vi "Tank Data Global.vi"(0 "Tank Data IN":dbl[](array[numeric]), 1 "Pump Data Mode":T4, 5 "Tank Temp Variables":T3, 7 "Watlow Present":bool, 9 "Pressure Offsets":dbl[](array[numeric])=[0.0, 0.0, 0.0, 0.0, 0.0, 0.0], 11 "Cal Coefficients":dbl[][](array[numeric]), 12 "Intitial Times":dbl[](array[numeric]), 13 "Pumps Present":bool[](array[boolean])) -> (4 "Tank Data OUT":dbl[](array[numeric]), 6 "Pump Data":T2={"Voltages"=[0.015201568603515625, 0.00335693359375, 0.003021240234375, 0.12260055541992188, 0.06085968017578125, 0.052234649658203125], "PumpCurrent"=[0.015201568603515625, 0.00335693359375, 0.003021240234375, 0.12260055541992188, 0.06085968017578125, 0.052234649658203125], "Speed"=[0.0, 0.0, 0.0, 0.0, 0.0, 0.0], "ControllerCurrent"=[0.015201568603515625, 0.00335693359375, 0.003021240234375, 0.12260055541992188, 0.06085968017578125, 0.052234649658203125], "Pressure"=[0.015201568603515625, 0.00335693359375, 0.003021240234375, 0.12260055541992188, 0.06085968017578125, 0.052234649658203125], "Flow"=[0.0, 0.0, 0.0, 0.125, 0.0625, 0.0625], "Elapsed Time (Display)"=[7.1, 7.1, 7.1, 458133.45, 458138.85000000003, 458126.75], "Avg Pressure"=0.0, "Avg Speed"=0.0, "Elapsed Time"=[4074.9003000000002, 4074.9003000000002, 4074.9003000000002, 4074.9003000000002, 4074.9003000000002, 4074.9003000000002]} {"Elapsed Time" format="%<%H:%M:%S>t"; "Elapsed Time (Display)" format="%<%H:%M:%S>t"; "Speed" format="%#_4f"; "ControllerCurrent" format="%#.1g"; "Pressure" format="%#.0f"; "Flow" format="%#.0f"; "PumpCurrent" format="%#.1g"; "Voltages" format="%#.0f"}, 8 "Tank Data":T1 {"PS Actual (V):" format="%.2f"; "Temp1" format="%#_2g"; "Temp2" format="%#_2g"}, 10 "Record Time (sec)":dbl)   [LabVIEW 2018]
uses:
  Type Defs/Pump Data Mode.ctl
  Controls/Tank Temp Variables.ctl
  Controls/Pump Data.ctl
  Controls/Tank Data.ctl
  <vilib>/ptbypt/NI_PtbyPt.lvlib
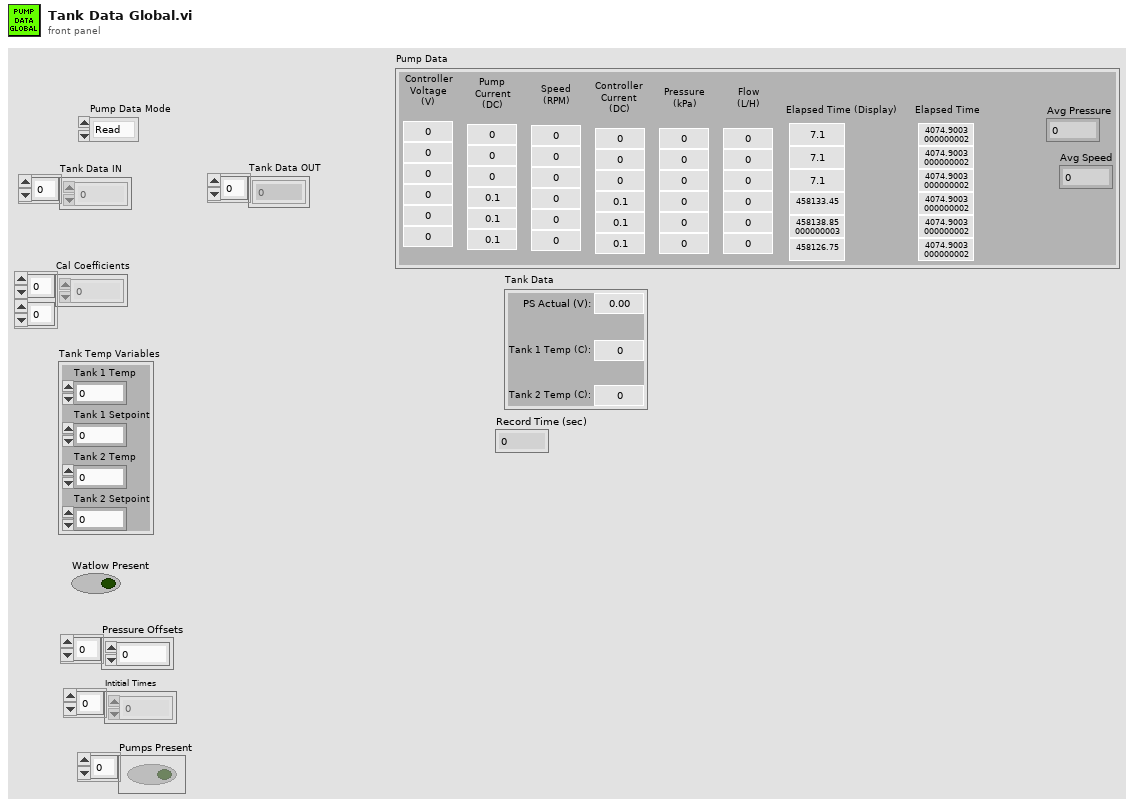
[diagram p1: front panel]
types:
  T1 = typedef "Tank Data.ctl" = cluster{"PS Actual (V):":dbl, "Temp1":dbl, "Temp2":dbl}
  T2 = typedef "Pump Data.ctl" = cluster{"Voltages":dbl[], "PumpCurrent":dbl[], "Speed":dbl[], "ControllerCurrent":dbl[], "Pressure":dbl[], "Flow":dbl[], "Elapsed Time (Display)":dbl[], "Avg Pressure":dbl, "Avg Speed":dbl, "Elapsed Time":dbl[]}
  T3 = typedef "Tank Temp Variables.ctl" = cluster{"Tank 1 Temp":sgl, "Tank 1 Setpoint":sgl, "Tank 2 Temp":sgl, "Tank 2 Setpoint":sgl}
  T4 = typedef "Pump Data Mode.ctl" = enum16{"Read", "Write Data", "Write Cal", "Write Watlow Data", "Write Pressure Offsets", "Write Initial Times", "Write Pumps Present"}
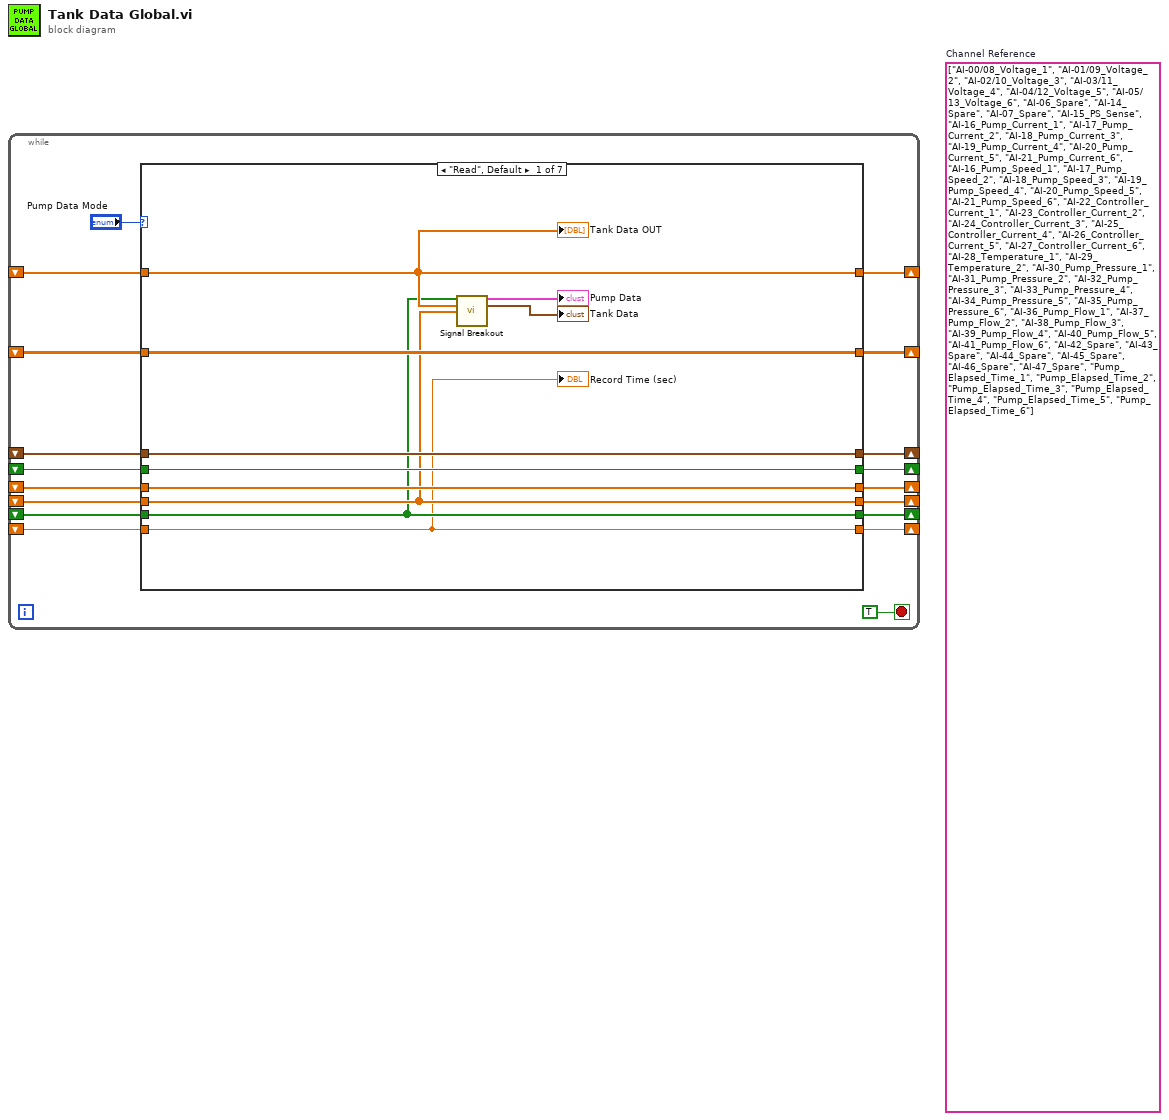
[diagram p0: block diagram]
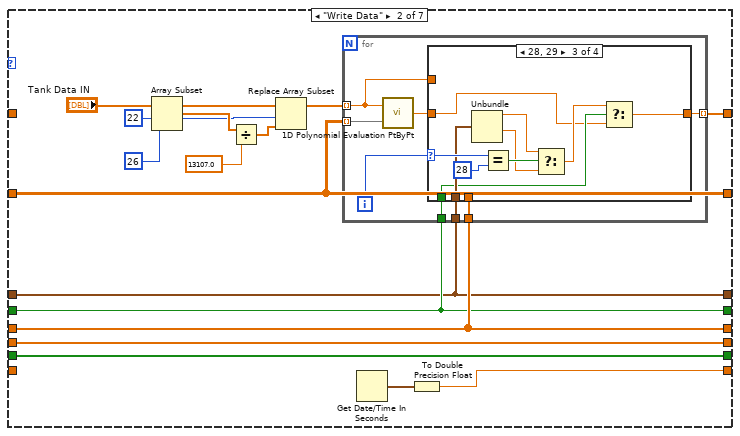
[diagram p2: hidden frame]
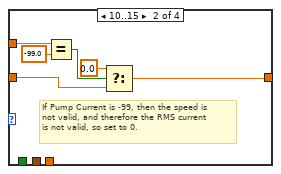
[diagram p4: hidden frame]
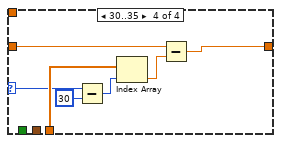
[diagram p5: hidden frame]
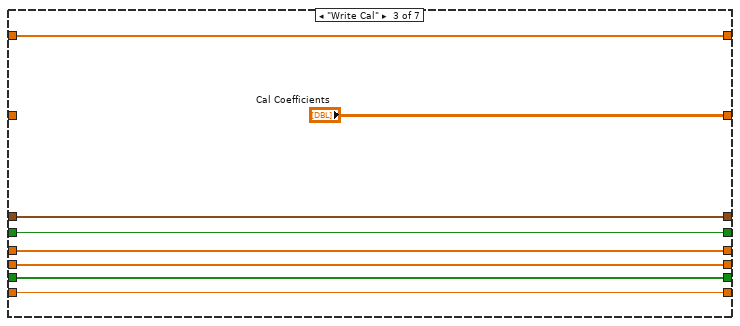
[diagram p6: hidden frame]
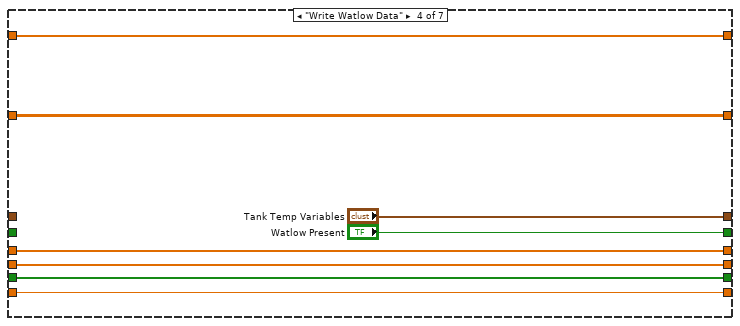
[diagram p7: hidden frame]
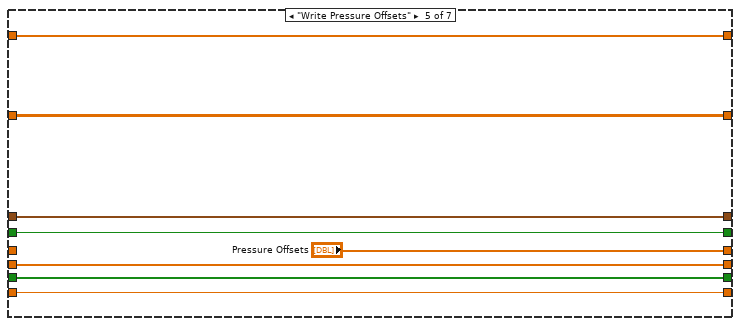
[diagram p8: hidden frame]
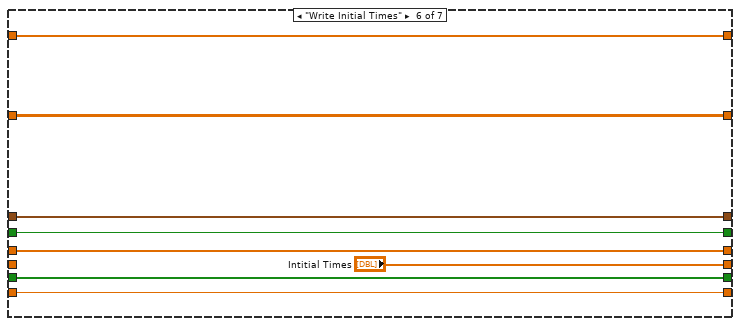
[diagram p9: hidden frame]
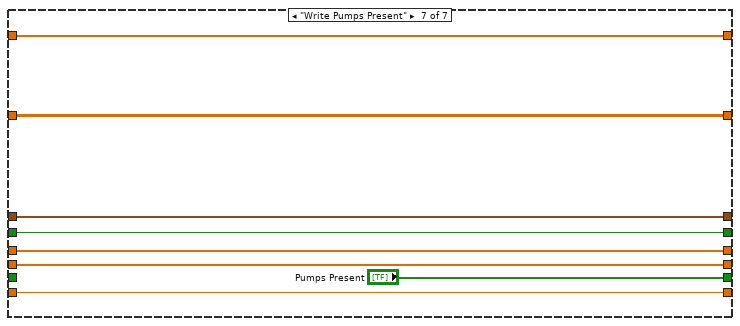
[diagram p10: hidden frame]
diagram:
  (unwired) string[] ["AI-00/08_Voltage_1", "AI-01/09_Voltage_2", "AI-02/10_Voltage_3", "AI-03/11_Voltage_4", "AI-04/12_Voltage_5", "AI-05/13_Voltage_6", "AI-06_Spare", "AI-14_Spare", "AI-07_Spare", "AI-15_PS_Sense", "AI-16_Pump_Current_1", "AI-17_Pump_Current_2", "AI-18_Pump_Current_3", "AI-19_Pump_Current_4", "AI-20_Pump_Current_5", "AI-21_Pump_Current_6", "AI-16_Pump_Speed_1", "AI-17_Pump_Speed_2", "AI-18_Pump_Speed_3", "AI-19_Pump_Speed_4", "AI-20_Pump_Speed_5", "AI-21_Pump_Speed_6", "AI-22_Controller_Current_1", "AI-23_Controller_Current_2", "AI-24_Controller_Current_3", "AI-25_Controller_Current_4", "AI-26_Controller_Current_5", "AI-27_Controller_Current_6", "AI-28_Temperature_1", "AI-29_Temperature_2", "AI-30_Pump_Pressure_1", "AI-31_Pump_Pressure_2", "AI-32_Pump_Pressure_3", "AI-33_Pump_Pressure_4", "AI-34_Pump_Pressure_5", "AI-35_Pump_Pressure_6", "AI-36_Pump_Flow_1", "AI-37_Pump_Flow_2", "AI-38_Pump_Flow_3", "AI-39_Pump_Flow_4", "AI-40_Pump_Flow_5", "AI-41_Pump_Flow_6", "AI-42_Spare", "AI-43_Spare", "AI-44_Spare", "AI-45_Spare", "AI-46_Spare", "AI-47_Spare", "Pump_Elapsed_Time_1", "Pump_Elapsed_Time_2", "Pump_Elapsed_Time_3", "Pump_Elapsed_Time_4", "Pump_Elapsed_Time_5", "Pump_Elapsed_Time_6"]  # Channel Reference
  n1 = while {
    shift-right: [w17] -> _
    shift-left: _ -> [w16]
    shift-right: [w14] -> _
    shift-left: _ -> [w13]
    shift-right: [w12] -> _
    shift-left: _ -> [w11]
    shift-right: [w10] -> _
    shift-left: _ -> [w8]
    shift-right: [w9] -> _
    shift-left: _ -> [w7]
    shift-right: [w6] -> _
    shift-left: _ -> [w5]
    shift-right: [w4] -> _
    shift-left: _ -> [w3]
    shift-right: [w2] -> _
    shift-left: _ -> [w1]
    stop <- TRUE stop-if-true
    n2 = case shown="\"Read\", Default" "Pump Data Mode" {
      tunnel: [w23 w44 w83 w90 w100 w108 w116] -> w17
      tunnel: w16 -> [w23 _ w83 w90 w100 w108 w116]
      tunnel: [w28 w43 "Cal Coefficients" w92 w99 w107 w115] -> w14
      tunnel: w13 -> [w28 w43 _ w92 w99 w107 w115]
      tunnel: [w27 w35 w82 w91 "Pressure Offsets" w104 w112] -> w12
      tunnel: w11 -> [w27 w35 w82 w91 _ w104 w112]
      tunnel: [w26 w33 w81 "Tank Temp Variables" w97 w106 w114] -> w10
      tunnel: [w25 w34 w80 "Watlow Present" w96 w105 w113] -> w9
      tunnel: w8 -> [w26 w33 w81 _ w97 w106 w114]
      tunnel: w7 -> [w25 w34 w80 _ w96 w105 w113]
      tunnel: [w24 w32 w79 w87 w95 "Intitial Times" w111] -> w6
      tunnel: w5 -> [w24 w32 w79 w87 w95 _ w111]
      tunnel: [w22 w31 w78 w86 w94 w102 "Pumps Present"] -> w4
      tunnel: w3 -> [w22 w31 w78 w86 w94 w102 _]
      tunnel: [w19 w29 w77 w85 w93 w101 w109] -> w2
      tunnel: w1 -> [w19 _ w77 w85 w93 w101 w109]
      frame "Read", Default {
        n3 = call "Signal Breakout.vi"("Pumps Enabled"=w22, "Tank Data"=w23, "Intitial Times"=w24) -> ("Pump Data"=→"Pump Data":T2, "Tank Data"=→"Tank Data":T1)  [unwired: 11 in]
        "Tank Data OUT" <- w23
        "Record Time (sec)" <- w19
      }
      frame "Write Data" {
        w38 = 22 ("index")
        n4 = Array Subset(array="Tank Data IN", index=w38, length=26) -> (w39:dbl[])
        n5 = Divide(x=w39, y=13107.0) -> (x/y=w41:dbl[])
        n6 = Replace Array Subset(array="Tank Data IN", new element=w41, index=w38) -> (w42:dbl[])
        n7 = for {
          tunnel: w43 -> [w52] mode=indexing
          tunnel: w42 -> [w48] mode=indexing
          tunnel: [w49] -> w44 mode=indexing
          tunnel: w35 -> [w47]
          tunnel: w34 -> [w46]
          tunnel: w33 -> [w45]
          i -> [w51]
          n8 = call <vilib>:"1D Polynomial Evaluation PtByPt.vi"("Coefficients: a"=w52, "x"=w48) -> ("y"=w50:dbl)
          n9 = case shown="28, 29" w51 {
            selector: w51 -> [_ _ w69 w75]
            tunnel: w50 -> [w53 w56 w61 w72]
            tunnel: [w53 w54 w60 w70] -> w49
            tunnel: w48 -> [_ w59 _ _]
            tunnel: w47 -> [_ _ _ w76]
            tunnel: w46 -> [_ _ w63 _]
            tunnel: w45 -> [_ _ w67 _]
            frame 0, Default {
            }
            frame 10..15 {
              # "If Pump Current is -99, then the speed is\nnot valid, and therefore the RMS current\nis not valid, so set to 0."
              n10 = Equal?(x=w59, y=-99.0) -> (x = y?=w57:bool)
              n11 = Select(t=0.0, s=w57, f=w56) -> (s? t:f=w54:dbl)
            }
            frame 28, 29 {
              n12 = Unbundle(w67) -> ("Tank 1 Temp"=w65:sgl, "Tank 2 Temp"=w64:sgl)  [unwired: 2 out]
              n13 = Equal?(x=w69, y=28) -> (x = y?=w66:bool)
              n14 = Select(t=w65, s=w66, f=w64) -> (s? t:f=w62:sgl)
              n15 = Select(t=w62, s=w63, f=w61) -> (s? t:f=w60:dbl)
            }
            frame 30..35 {
              n16 = Subtract(x=w75, y=30) -> (x-y=w73:i32)
              n17 = Index Array(array=w76, index=w73) -> (element=w71:dbl)
              n18 = Subtract(x=w72, y=w71) -> (x-y=w70:dbl)
            }
          }
        }
        n19 = Get Date/Time In Seconds() -> (seconds since 1Jan1904=w30:timestamp)
        n20 = To Double Precision Float(number=w30) -> (double precision float=w29:dbl)
      }
      frame "Write Cal" {
      }
      frame "Write Watlow Data" {
      }
      frame "Write Pressure Offsets" {
      }
      frame "Write Initial Times" {
      }
      frame "Write Pumps Present" {
      }
    }
  }
